vi "control daq.vi"(0 "Camera Device  IN":T1, 1 "Image Device IN":cluster{"Image":T5, "errorImage":errorcluster}, 2 "DAQ Device IN":T3={"DAQ Fs (S/s)"=10000.0, "task"="", "error"={"status"=FALSE, "code"=0, "source"=""}, "Min Value"=-10.0, "Max Value"=10.0}, 3 "Time Control Parameters":cluster{"# samples":u32, "tiempos (ms)":dbl}, 4 "Parametros Maximos":T6, 5 "detla Parametros":T6, 6 "Camara ON?":bool, 7 "Control Parameters":T4={"N Init Avg"=6, "N Avg Best"=3, "% Best to test"=0.95, "% Best to beat"=1.0}, 8 "Control?":bool=TRUE, 9 "Reset Control":bool, 10 "Ajuste?":bool=TRUE, 11 "Calibracion DAQ":T2) -> (14 "Camera Device OUT":T1, 15 "Image Device OUT":cluster{"Image":T5, "errorImage":errorcluster}, 16 "DAQ Device OUT":T3={"DAQ Fs (S/s)"=0.0, "task"="", "error"={"status"=FALSE, "code"=0, "source"=""}, "Min Value"=-10.0, "Max Value"=10.0}, 17 "Contraste":dbl, 18 "Waveform":waveform(dbl), 19 "Señal de Control":dbl[](array[numeric]))   [LabVIEW 2010]
uses:
  <vilib>/vision/Image Controls.llb/IMAQ Image.ctl
  <vilib>/measure/NI_MABase.lvlib
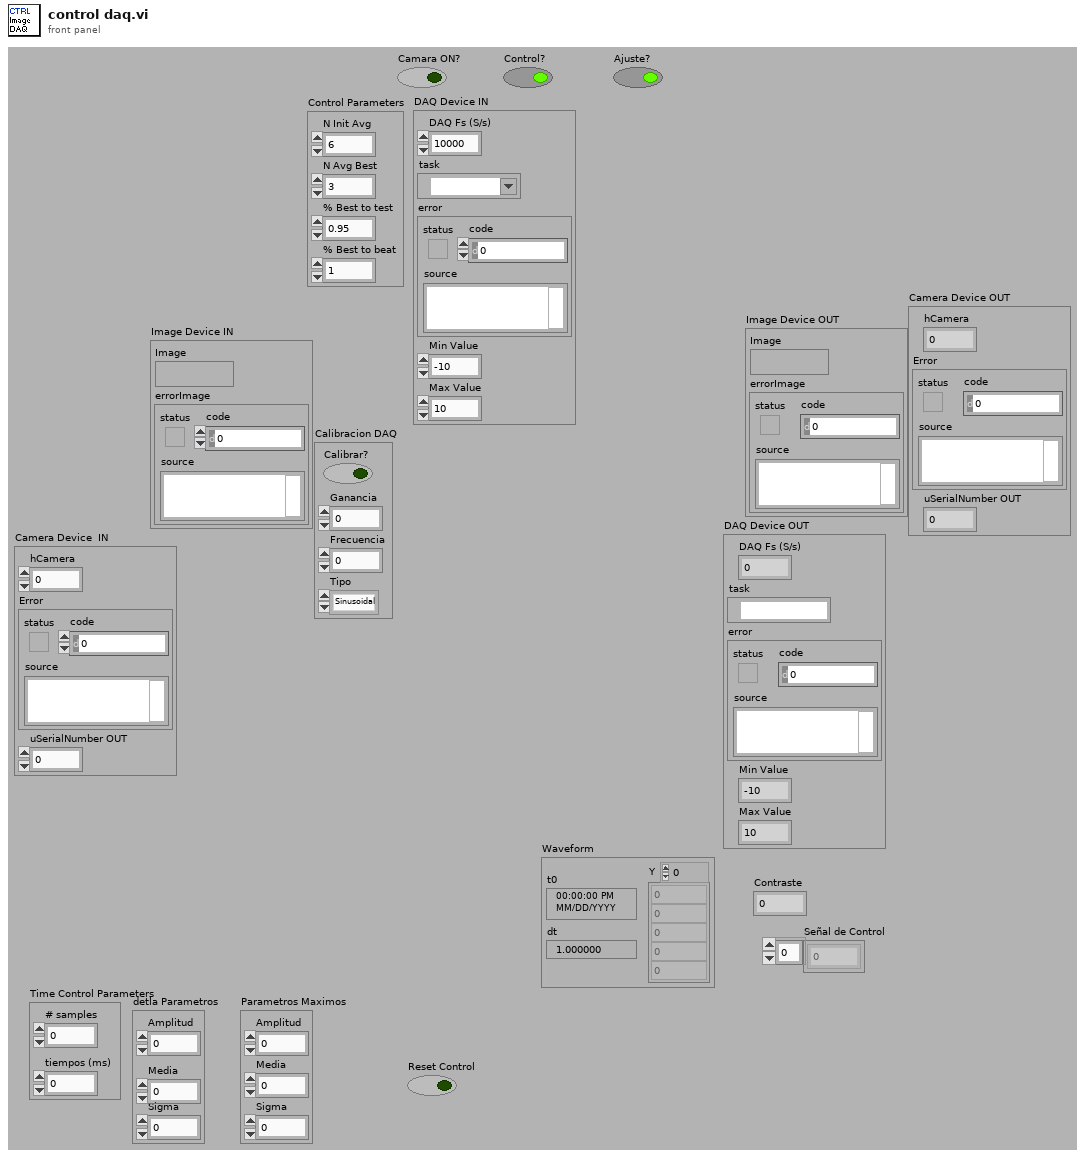
[diagram p1: front panel]
types:
  T1 = cluster{"hCamera":u32, "Error":errorcluster, "uSerialNumber OUT":u32}
  T2 = cluster{"Calibrar?":bool, "Ganancia":dbl, "Frecuencia":dbl, "Tipo":enum16{"Sinusoidal", "Triangular", "Cuadrada"}}
  T3 = cluster{"DAQ Fs (S/s)":dbl, "task":refnum<k21>, "error":errorcluster, "Min Value":dbl, "Max Value":dbl}
  T4 = cluster{"N Init Avg":u32, "N Avg Best":u32, "% Best to test":dbl, "% Best to beat":dbl}
  T5 = typedef "IMAQ Image.ctl" = refnum<image>
  T6 = cluster{"Amplitud":dbl, "Media":dbl, "Sigma":dbl}
  T7 = cluster{"DAQ Limits":cluster{"max":dbl, "min":dbl}, "Control Limits":cluster{"max":dbl, "min":dbl}}
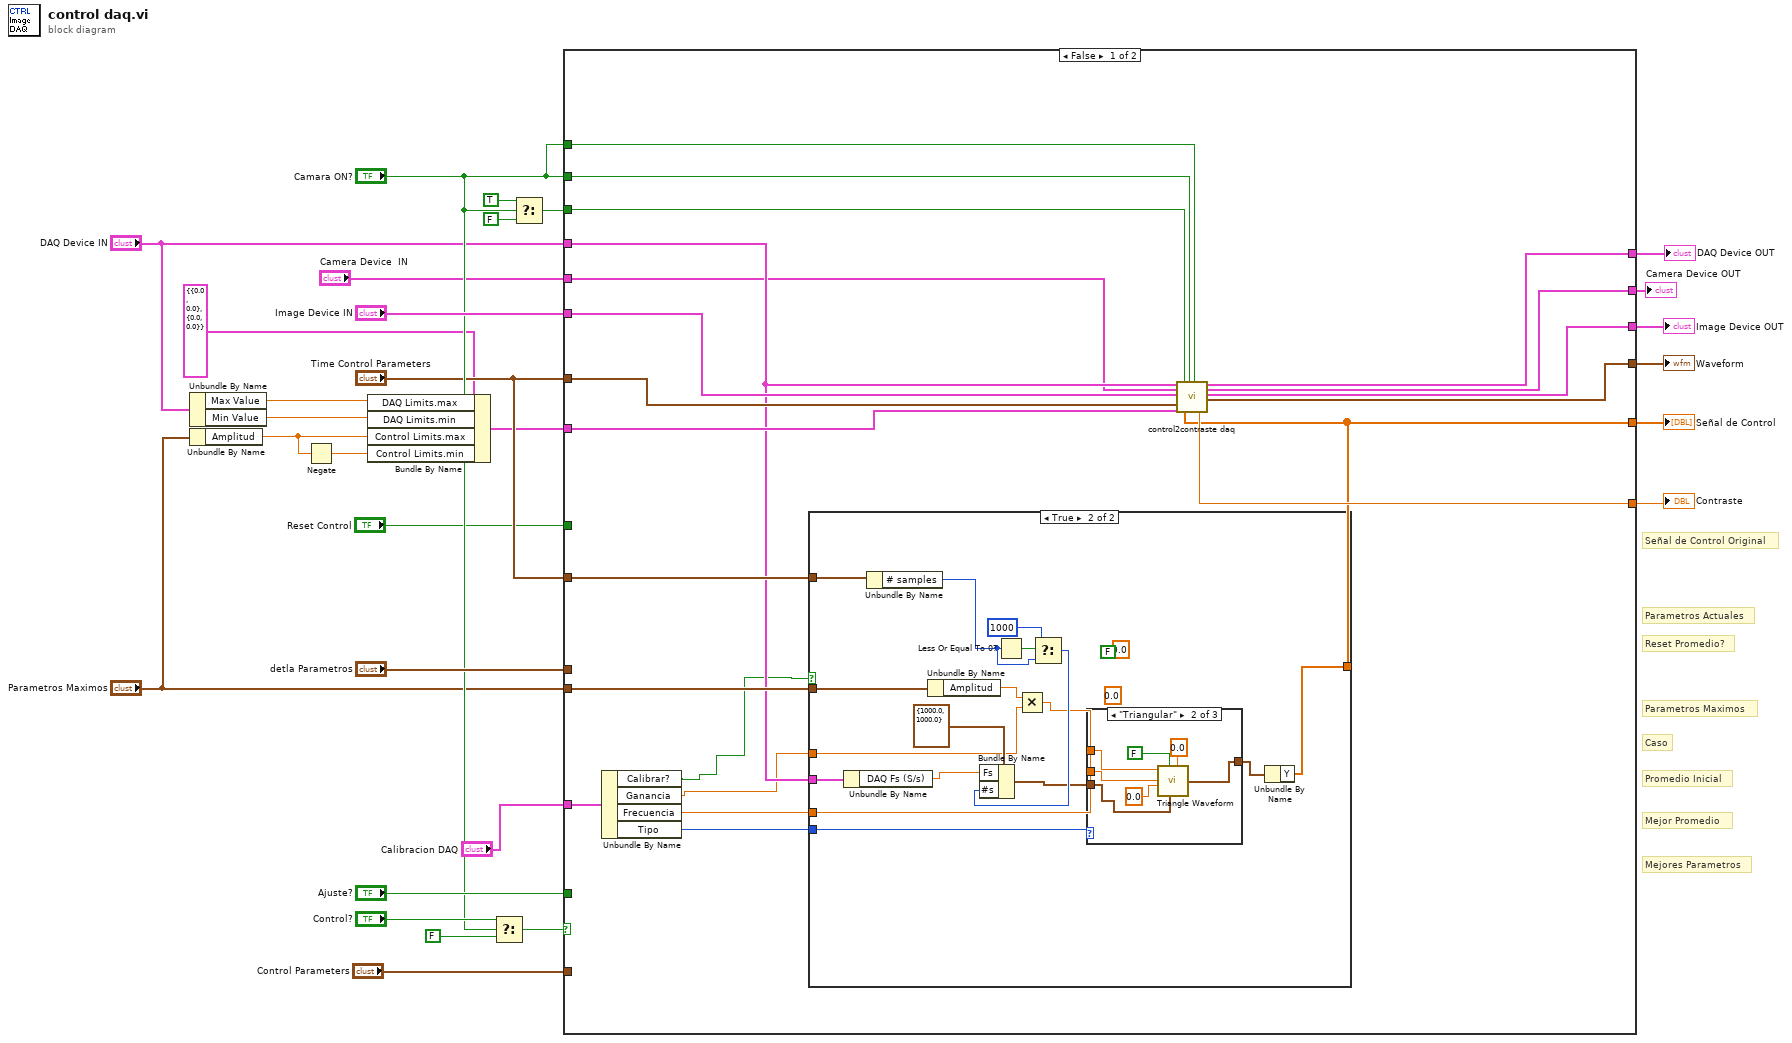
[diagram p0: block diagram]
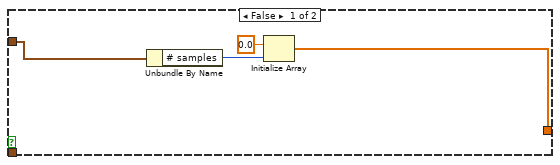
[diagram p2: hidden frame]
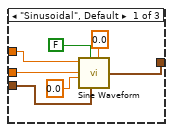
[diagram p3: hidden frame]
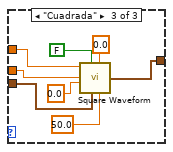
[diagram p4: hidden frame]
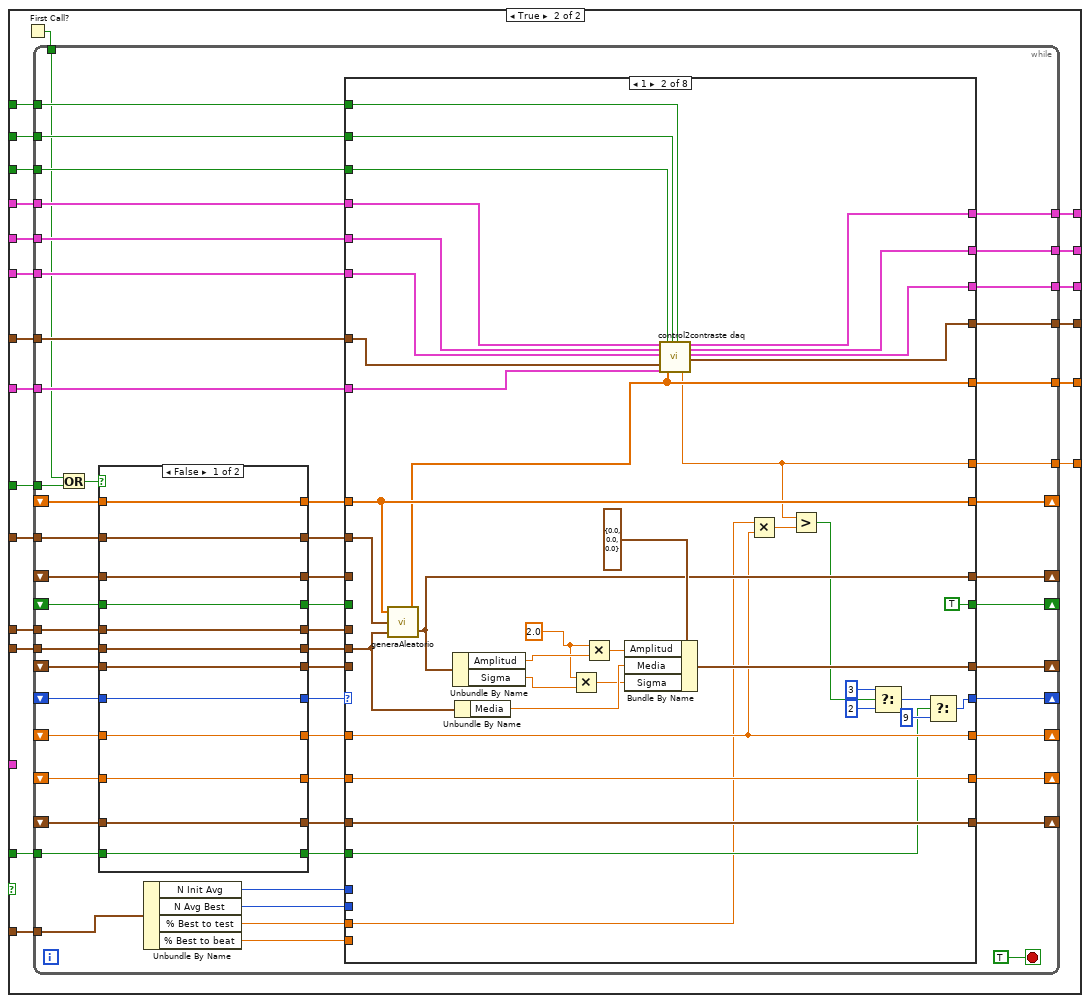
[diagram p5: hidden frame]
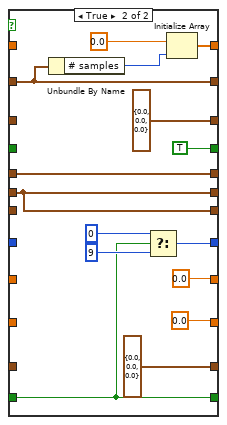
[diagram p6: hidden frame]
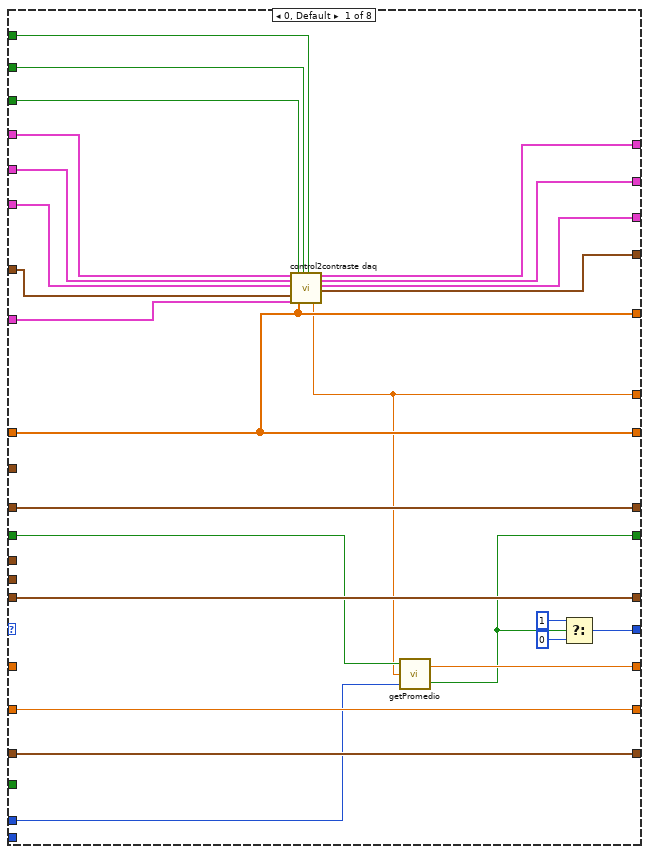
[diagram p7: hidden frame]
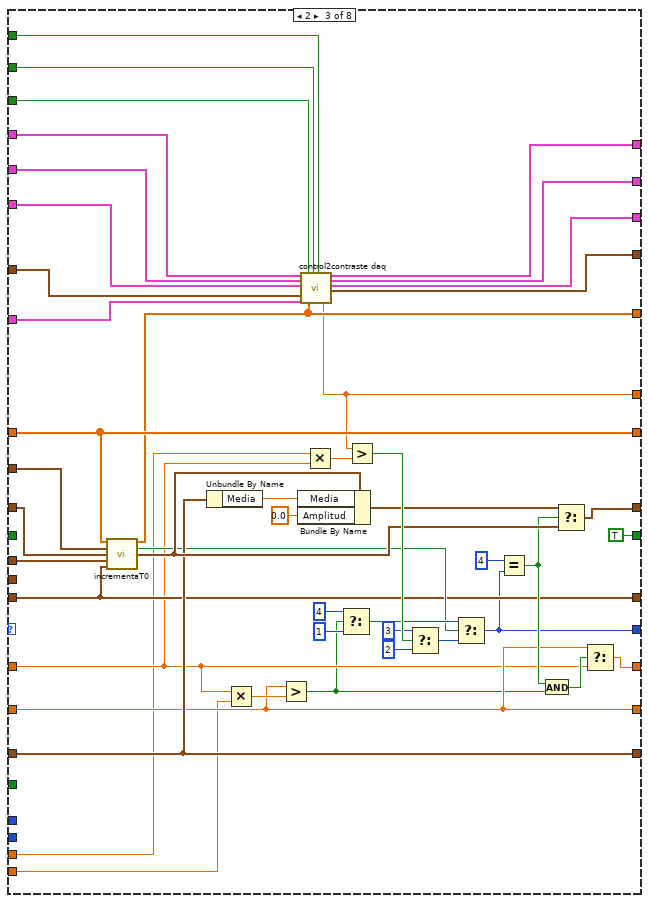
[diagram p8: hidden frame]
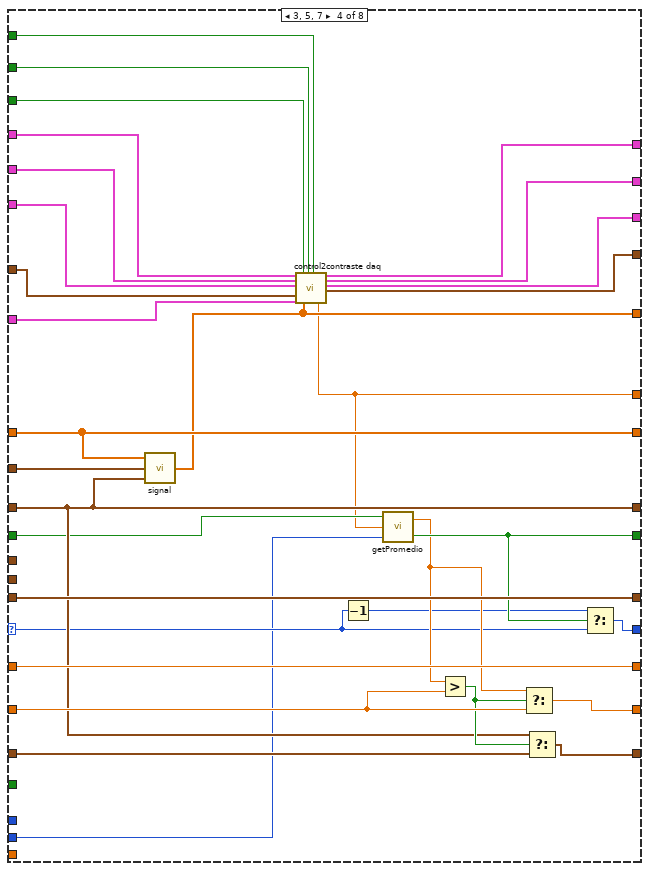
[diagram p9: hidden frame]
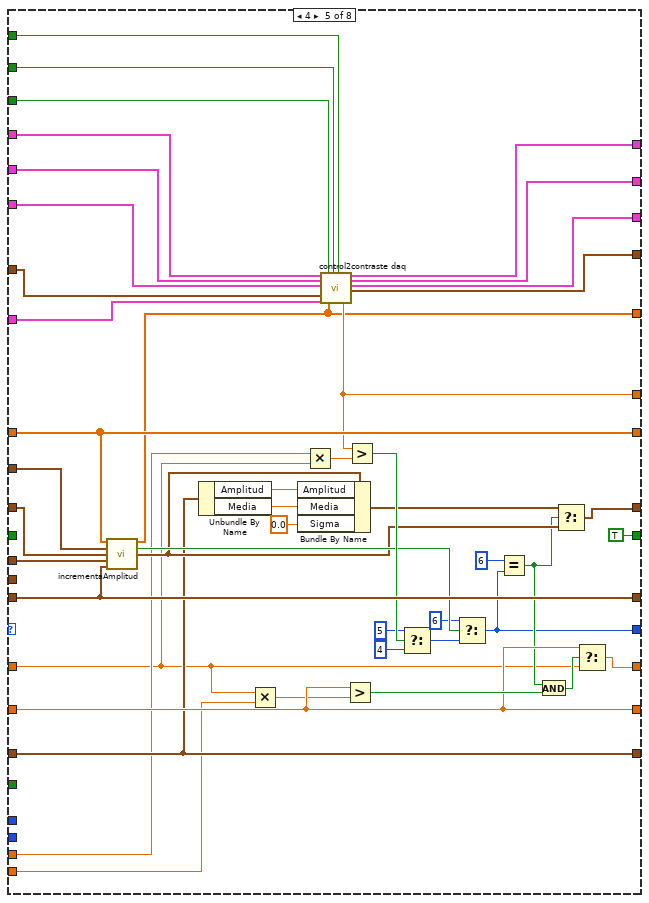
[diagram p10: hidden frame]
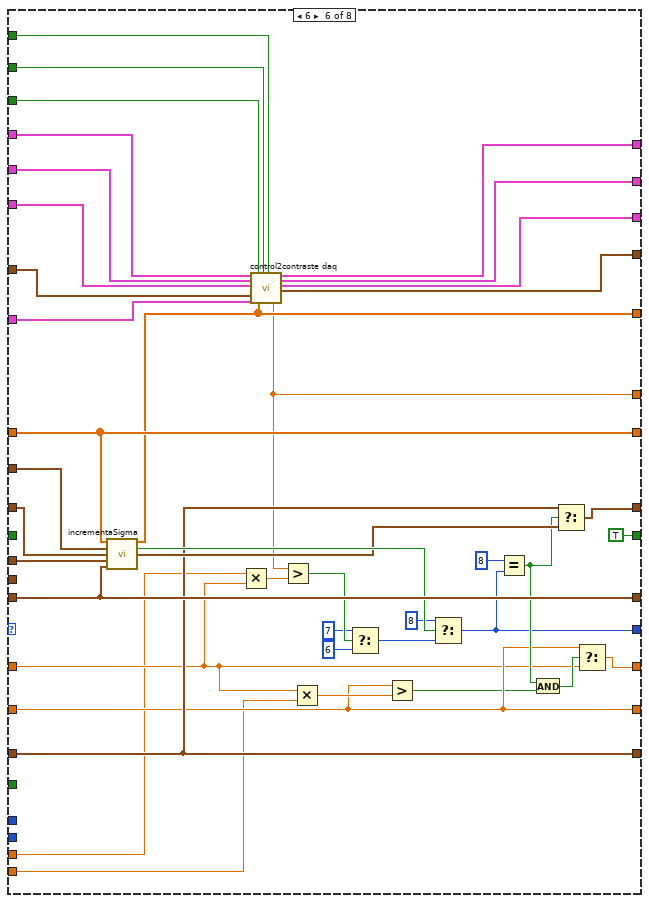
[diagram p11: hidden frame]
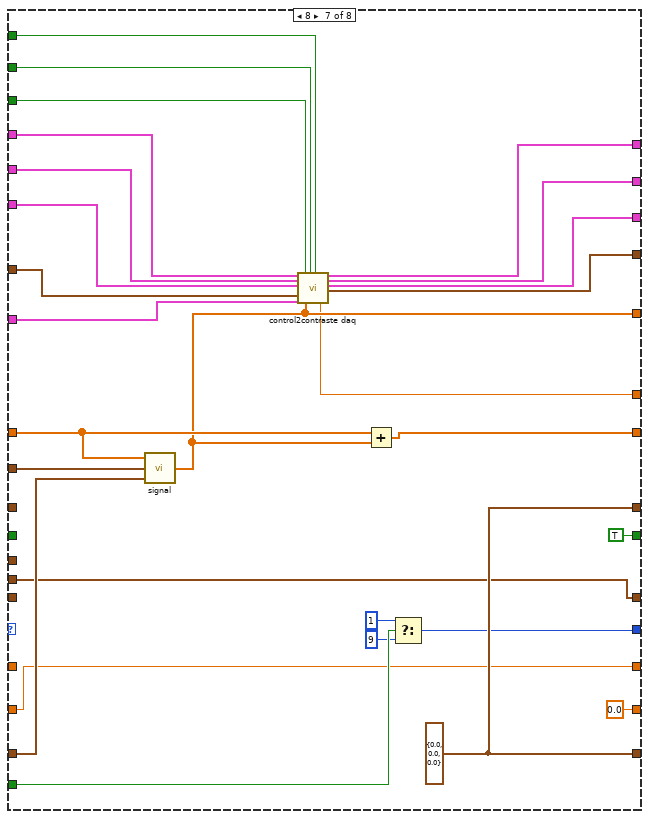
[diagram p12: hidden frame]
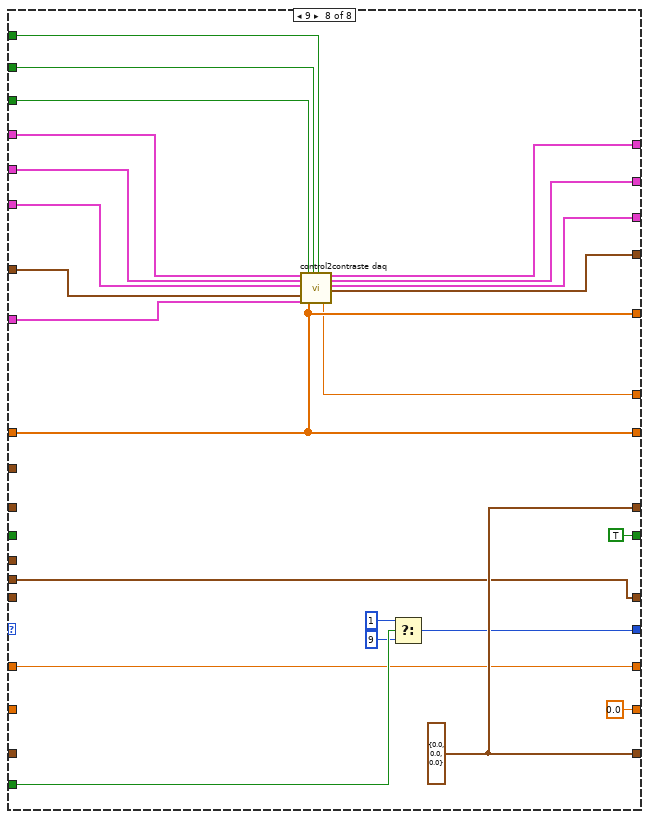
[diagram p13: hidden frame]
diagram:
  # "Reset Promedio?"
  # "Mejores Parametros"
  # "Mejor Promedio"
  # "Señal de Control Original"
  # "Parametros Actuales"
  # "Parametros Maximos"
  # "Caso"
  # "Promedio Inicial"
  n1 = Unbundle By Name("DAQ Device IN") -> ("Max Value"=w9:dbl, "Min Value"=w8:dbl)
  n2 = Unbundle By Name("Parametros Maximos") -> ("Amplitud"=w6:dbl)
  n3 = Negate(x=w6) -> (-x=w7:dbl)
  n4 = Bundle By Name(cluster=T7 {"DAQ Limits"={"max"=0.0, "min"=0.0}, "Control Limits"={"max"=0.0, "min"=0.0}} ("Limites"), "DAQ Limits.max"=w9, "DAQ Limits.min"=w8, "Control Limits.max"=w6, "Control Limits.min"=w7) -> (w10:T7)
  n5 = Select(t="Control?", s="Camara ON?", f=FALSE) -> (s? t:f=w19:bool)
  n6 = Select(t=TRUE, s="Camara ON?", f=FALSE) -> (s? t:f=w22:bool)
  n7 = case shown="False" w19 {
    tunnel: "Time Control Parameters" -> [w50 w114]
    tunnel: "detla Parametros" -> [_ w113]
    tunnel: "Parametros Maximos" -> [w38 w112]
    tunnel: "Ajuste?" -> [_ w110]
    tunnel: [w36 w109] -> w27
    tunnel: [w49 w108] -> w26
    tunnel: w10 -> [w48 w107]
    tunnel: "Time Control Parameters" -> [w47 w106]
    tunnel: "Image Device IN" -> [w46 w105]
    tunnel: "Camera Device  IN" -> [w30 w104]
    tunnel: "DAQ Device IN" -> [w37 w103]
    tunnel: w22 -> [w45 w102]
    tunnel: "Camara ON?" -> [w44 w101]
    tunnel: "Camara ON?" -> [w43 w100]
    tunnel: [w42 w99] -> w24
    tunnel: [w41 w98] -> w23
    tunnel: [w40 w97] -> w1
    tunnel: [w39 w96] -> w12
    tunnel: "Reset Control" -> [_ w95]
    tunnel: "Control Parameters" -> [_ w94]
    tunnel: "Calibracion DAQ" -> [w31 _]
    frame False {
      n8 = Unbundle By Name(w31) -> ("Calibrar?"=w35:bool, "Ganancia"=w34:dbl, "Frecuencia"=w33:dbl, "Tipo"=w32:enum16{"Sinusoidal", "Triangular", "Cuadrada"})
      n9 = case shown="True" w35 {
        tunnel: w50 -> [w52 w63]
        tunnel: w38 -> [_ w71]
        tunnel: w37 -> [_ w69]
        tunnel: [w51 w62] -> w36
        tunnel: w34 -> [_ w61]
        tunnel: w33 -> [_ w56]
        tunnel: w32 -> [_ w59]
        frame False {
          n10 = Unbundle By Name(w52) -> ("# samples"=w53:u32)
          n11 = Initialize Array(0.0 ("element"), w53) -> (w51:dbl[])
        }
        frame True {
          (unwired) FALSE ("reset signal")
          (unwired) 0.0 ("offset")
          (unwired) 0.0 ("phase")
          n12 = Unbundle By Name(w69) -> ("DAQ Fs (S/s)"=w68:dbl)
          n13 = Unbundle By Name(w63) -> ("# samples"=w64:u32)
          n14 = Unbundle By Name(w71) -> ("Amplitud"=w60:dbl)
          n15 = Less Or Equal To 0?(x=w64) -> (x <= 0?=w67:bool)
          n16 = Multiply(x=w60, y=w61) -> (x*y=w57:dbl)
          n17 = Select(t=u32 1000, s=w67, f=w64) -> (s? t:f=w65:u32)
          n18 = Bundle By Name(cluster=cluster{"Fs":dbl, "#s":dbl} {"Fs"=1000.0, "#s"=1000.0} ("sampling info"), "Fs"=w68, "#s"=w65) -> (w58:cluster{"Fs":dbl, "#s":dbl})
          n19 = case shown="\"Triangular\"" w59 {
            tunnel: w58 -> [w78 w80 w90]
            tunnel: w57 -> [w76 w81 w89]
            tunnel: w56 -> [w75 w82 w88]
            tunnel: [w72 w79 w87] -> w55
            frame "Sinusoidal", Default {
              n20 = call <vilib>:"Sine Waveform.vi"("offset"=0.0, "sampling info"=w78, "reset signal"=FALSE, "phase"=0.0, "amplitude"=w76, "frequency"=w75) -> ("signal out"=w72:waveform(dbl))  [unwired: 4 in, 1 out]
            }
            frame "Triangular" {
              n21 = call <vilib>:"Triangle Waveform.vi"("offset"=0.0, "sampling info"=w80, "reset signal"=FALSE, "phase"=0.0, "amplitude"=w81, "frequency"=w82) -> ("signal out"=w79:waveform(dbl))  [unwired: 4 in, 1 out]
            }
            frame "Cuadrada" {
              n22 = call <vilib>:"Square Waveform.vi"("duty cycle (%)"=50.0, "offset"=0.0, "sampling info"=w90, "reset signal"=FALSE, "phase"=0.0, "amplitude"=w89, "frequency"=w88) -> ("signal out"=w87:waveform(dbl))  [unwired: 3 in, 1 out]
            }
          }
          n23 = Unbundle By Name(w55) -> ("Y"=w62:dbl[])
        }
      }
      n24 = call "control2contraste daq.vi"("DAQ Device IN"=w37, "Camera Device  IN"=w30, "Image Device IN"=w46, "Time Control Parameters"=w47, "Limites"=w48, "DAQ?"=w45, "ControlSignal"=w36, "Streeam?"=w44, "Mostrar?"=w43) -> ("Contraste"=w49:dbl, "DAQ Device OUT"=w39:T3, "Camera Device OUT"=w40:T1, "Image Device OUT"=w41:cluster{"Image":T5, "errorImage":errorcluster}, "Waveform"=w42:waveform(dbl))  [unwired: 6 in]
    }
    frame True {
      n25 = First Call?() -> (First Call?: T/F=w111:bool)
      n26 = while {
        shift-right: [w166] -> _
        shift-left: _ -> [w153]
        tunnel: w114 -> [w145]
        shift-right: [w169] -> _
        shift-left: _ -> [w161]
        shift-right: [w168] -> _
        shift-left: _ -> [w155]
        shift-right: [w167] -> _
        shift-left: _ -> [w159]
        shift-right: [w165] -> _
        shift-left: _ -> [w151]
        tunnel: w113 -> [w142]
        shift-right: [w164] -> _
        shift-left: _ -> [w149]
        shift-right: [w163] -> _
        shift-left: _ -> [w147]
        shift-right: [w162] -> _
        shift-left: _ -> [w157]
        tunnel: w110 -> [w144]
        tunnel: w112 -> [w143]
        tunnel: w111 -> [w122]
        tunnel: [w137] -> w109
        tunnel: [w136] -> w108
        tunnel: w107 -> [w135]
        tunnel: w106 -> [w134]
        tunnel: w105 -> [w133]
        tunnel: w104 -> [w132]
        tunnel: w103 -> [w131]
        tunnel: w102 -> [w130]
        tunnel: w101 -> [w129]
        tunnel: w100 -> [w128]
        tunnel: [w127] -> w99
        tunnel: [w126] -> w98
        tunnel: [w125] -> w97
        tunnel: [w124] -> w96
        tunnel: w95 -> [w120]
        tunnel: w94 -> [w119]
        stop <- TRUE stop-if-true
        n27 = Or(x=w122, y=w120) -> (x .or. y?=w121:bool)
        n28 = case shown="False" w121 {
          tunnel: w161 -> [w181 _]
          tunnel: [w181 w196] -> w160
          tunnel: [w180 T6 {"Amplitud"=0.0, "Media"=0.0, "Sigma"=0.0} ("Parametros Iniciales")] -> w158
          tunnel: w159 -> [w180 _]
          tunnel: w157 -> [w179 _]
          tunnel: [w179 TRUE] -> w156
          tunnel: w155 -> [w178 _]
          tunnel: [w178 w185] -> w154
          tunnel: w153 -> [w177 _]
          tunnel: [w177 w186] -> w152
          tunnel: w151 -> [w176 _]
          tunnel: [w176 0.0 ("Contraste Promedio")] -> w150
          tunnel: w149 -> [w175 _]
          tunnel: [w175 0.0 ("Contraste Promedio")] -> w148
          tunnel: w147 -> [w174 _]
          tunnel: [w174 T6 {"Amplitud"=0.0, "Media"=0.0, "Sigma"=0.0} ("Parametros Maximos")] -> w146
          tunnel: w145 -> [w173 w182]
          tunnel: w143 -> [w171 w185]
          tunnel: w144 -> [w170 w183]
          tunnel: [w171 w185] -> w141
          tunnel: [w172 w184] -> w140
          tunnel: w142 -> [w172 w184]
          tunnel: [w170 w183] -> w139
          tunnel: [w173 w182] -> w138
          frame False {
          }
          frame True {
            n29 = Unbundle By Name(w182) -> ("# samples"=w194:u32)
            n30 = Select(t=u32 0, s=w183, f=u32 9) -> (s? t:f=w186:u32)
            n31 = Initialize Array(0.0 ("element"), w194) -> (w196:dbl[])
          }
        }
        n32 = Unbundle By Name(w119) -> ("N Init Avg"=w118:u32, "N Avg Best"=w117:u32, "% Best to test"=w116:dbl, "% Best to beat"=w115:dbl)
        n33 = case shown="1" w152 {
          selector: w152 -> [_ _ _ w322 _ _ _ _]
          tunnel: w160 -> [w211 w259 w303 w336 w379 w420 w442 w464]
          tunnel: w138 -> [_ w260 w306 w337 w382 w423 w450 _]
          tunnel: w154 -> [w214 _ w285 w328 w378 w419 _ _]
          tunnel: [w211 w259 w303 w336 w379 w420 w441 w464] -> w169
          tunnel: [w214 w258 w285 w328 w378 w419 w438 w466] -> w168
          tunnel: [w215 w256 w293 w327 w368 w411 w447 w472] -> w167
          tunnel: [w221 w223 w268 w335 w345 w389 w439 w467] -> w166
          tunnel: [w216 w246 w297 w334 w373 w415 w440 w465] -> w165
          tunnel: w150 -> [_ w246 w263 w334 w338 w385 _ w465]
          tunnel: [w210 w224 w283 w320 w359 w405 w436 w463] -> w136
          tunnel: [w211 w240 w284 w321 w358 w406 w437 w464] -> w137
          tunnel: w158 -> [w215 _ w305 w327 w381 w422 _ _]
          tunnel: w140 -> [_ _ w304 _ w380 w421 _ _]
          tunnel: [w217 w249 w265 w333 w371 w387 0.0 ("Contraste Promedio") 0.0 ("Contraste Promedio")] -> w164
          tunnel: [w218 w248 w290 w331 w365 w407 w447 w472] -> w163
          tunnel: w146 -> [w218 w248 w290 w329 w365 w407 w449 _]
          tunnel: w148 -> [w217 w249 w265 w332 w371 w387 w440 _]
          tunnel: w156 -> [w212 _ _ w326 _ _ _ _]
          tunnel: [w213 TRUE ("Llego a N?") TRUE ("Llego a N?") w325 TRUE ("Llego a N?") TRUE ("Llego a N?") TRUE ("Llego a N?") TRUE ("Llego a N?")] -> w162
          tunnel: w139 -> [_ w225 _ _ _ _ w445 w470]
          tunnel: w141 -> [_ w241 _ _ _ _ w438 w466]
          tunnel: w135 -> [w209 w239 w282 w319 w342 w404 w435 w462]
          tunnel: w134 -> [w208 w238 w281 w318 w343 w400 w434 w461]
          tunnel: w133 -> [w207 w237 w280 w317 w357 w399 w433 w460]
          tunnel: w132 -> [w206 w236 w279 w316 w356 w398 w432 w459]
          tunnel: w131 -> [w205 w228 w278 w315 w344 w397 w431 w458]
          tunnel: w130 -> [w204 w235 w277 w314 w355 w401 w430 w457]
          tunnel: w129 -> [w203 w234 w276 w313 w354 w402 w429 w456]
          tunnel: w128 -> [w202 w233 w275 w312 w353 w403 w428 w455]
          tunnel: [w201 w232 w274 w311 w352 w396 w427 w454] -> w127
          tunnel: [w200 w230 w273 w310 w351 w395 w426 w453] -> w126
          tunnel: [w199 w231 w272 w309 w350 w394 w425 w452] -> w125
          tunnel: [w198 w229 w271 w308 w349 w393 w424 w451] -> w124
          tunnel: w118 -> [w197 _ _ _ _ _ _ _]
          tunnel: w117 -> [_ _ _ w307 _ _ _ _]
          tunnel: w116 -> [_ w222 w261 _ w341 w384 _ _]
          tunnel: w115 -> [_ _ w264 _ w340 w386 _ _]
          frame 0, Default {
            n34 = call "control2contraste daq.vi"("DAQ Device IN"=w205, "Camera Device  IN"=w206, "Image Device IN"=w207, "Time Control Parameters"=w208, "Limites"=w209, "DAQ?"=w204, "ControlSignal"=w211, "Streeam?"=w203, "Mostrar?"=w202) -> ("Contraste"=w210:dbl, "DAQ Device OUT"=w198:T3, "Camera Device OUT"=w199:T1, "Image Device OUT"=w200:cluster{"Image":T5, "errorImage":errorcluster}, "Waveform"=w201:waveform(dbl))  [unwired: 6 in]
            n35 = call "getPromedio.vi"("N"=w197, "Contraste"=w210, "Reset"=w212) -> ("Llego a N?"=w213:bool, "Contraste Promedio"=w216:dbl)
            n36 = Select(t=u32 1, s=w213, f=u32 0) -> (s? t:f=w221:u32)
          }
          frame 1 {
            w251 = 2.0 ("x")
            n37 = call "generaAleatorio.vi"("Parametros Maximos"=w241, "Sound Parameters"=w260, "Señal de Control IN"=w259) -> ("Parametros Iniciales"=w256:T6, "Out"=w240:dbl[])
            n38 = Unbundle By Name(w256) -> ("Amplitud"=w255:dbl, "Sigma"=w252:dbl)
            n39 = Unbundle By Name(w241) -> ("Media"=w253:dbl)
            n40 = Multiply(x=w251, y=w252) -> (x*y=w250:dbl)
            n41 = Multiply(x=w251, y=w255) -> (x*y=w254:dbl)
            n42 = Bundle By Name(cluster=T6 {"Amplitud"=0.0, "Media"=0.0, "Sigma"=0.0} ("Parametros Iniciales"), "Amplitud"=w254, "Media"=w253, "Sigma"=w250) -> (w258:T6)
            n43 = call "control2contraste daq.vi"("DAQ Device IN"=w228, "Camera Device  IN"=w236, "Image Device IN"=w237, "Time Control Parameters"=w238, "Limites"=w239, "DAQ?"=w235, "ControlSignal"=w240, "Streeam?"=w234, "Mostrar?"=w233) -> ("Contraste"=w224:dbl, "DAQ Device OUT"=w229:T3, "Camera Device OUT"=w231:T1, "Image Device OUT"=w230:cluster{"Image":T5, "errorImage":errorcluster}, "Waveform"=w232:waveform(dbl))  [unwired: 6 in]
            n44 = Multiply(x=w222, y=w246) -> (x*y=w247:dbl)
            n45 = Greater?(x=w224, y=w247) -> (0:w245:bool)
            n46 = Select(t=u32 3, s=w245, f=u32 2) -> (s? t:f=w226:u32)
            n47 = Select(t=w226, s=w225, f=u32 9) -> (s? t:f=w223:u32)
          }
          frame 2 {
            n48 = call "incrementaT0.vi"("Señal de Control IN"=w303, "Sound Parameters"=w306, "Parametros Actuales IN"=w305, "detla Parametros"=w304, "Parametros Maximos"=w285) -> ("Out"=w284:dbl[], "Tope?"=w287:bool, "Parametros Actuales OUT"=w291:T6)  [unwired: 8 in]
            n49 = Unbundle By Name(w290) -> ("Media"=w289:dbl)
            n50 = Multiply(x=w263, y=w264) -> (x*y=w266:dbl)
            n51 = Greater?(x=w265, y=w266) -> (0:w262:bool)
            n52 = Bundle By Name(cluster=w291, "Media"=w289, "Amplitud"=0.0) -> (w292:T6)
            n53 = call "control2contraste daq.vi"("DAQ Device IN"=w278, "Camera Device  IN"=w279, "Image Device IN"=w280, "Time Control Parameters"=w281, "Limites"=w282, "DAQ?"=w277, "ControlSignal"=w284, "Streeam?"=w276, "Mostrar?"=w275) -> ("Contraste"=w283:dbl, "DAQ Device OUT"=w271:T3, "Camera Device OUT"=w272:T1, "Image Device OUT"=w273:cluster{"Image":T5, "errorImage":errorcluster}, "Waveform"=w274:waveform(dbl))  [unwired: 6 in]
            n54 = Multiply(x=w261, y=w263) -> (x*y=w302:dbl)
            n55 = Select(t=u32 4, s=w262, f=u32 1) -> (s? t:f=w298:u32)
            n56 = Greater?(x=w283, y=w302) -> (0:w301:bool)
            n57 = Select(t=u32 3, s=w301, f=u32 2) -> (s? t:f=w267:u32)
            n58 = Select(t=w298, s=w287, f=w267) -> (s? t:f=w268:u32)
            n59 = Equal?(x=u32 4, y=w268) -> (x = y?=w286:bool)
            n60 = And(x=w286, y=w262) -> (x .and. y?=w296:bool)
            n61 = Select(t=w292, s=w286, f=w291) -> (s? t:f=w293:T6)
            n62 = Select(t=w265, s=w296, f=w263) -> (s? t:f=w297:dbl)
          }
          frame 3, 5, 7 {
            n63 = call "signal.vi"("Parametros Actuales IN"=w327, "Sound Parameters"=w337, "Señal de Control IN"=w336) -> ("Out"=w321:dbl[])
            n64 = call "control2contraste daq.vi"("DAQ Device IN"=w315, "Camera Device  IN"=w316, "Image Device IN"=w317, "Time Control Parameters"=w318, "Limites"=w319, "DAQ?"=w314, "ControlSignal"=w321, "Streeam?"=w313, "Mostrar?"=w312) -> ("Contraste"=w320:dbl, "DAQ Device OUT"=w308:T3, "Camera Device OUT"=w309:T1, "Image Device OUT"=w310:cluster{"Image":T5, "errorImage":errorcluster}, "Waveform"=w311:waveform(dbl))  [unwired: 6 in]
            n65 = Decrement(x=w322) -> (x-1=w323:u32)
            n66 = call "getPromedio.vi"("N"=w307, "Contraste"=w320, "Reset"=w326) -> ("Llego a N?"=w325:bool, "Contraste Promedio"=w324:dbl)
            n67 = Greater?(x=w324, y=w332) -> (0:w330:bool)
            n68 = Select(t=w324, s=w330, f=w332) -> (s? t:f=w333:dbl)
            n69 = Select(t=w327, s=w330, f=w329) -> (s? t:f=w331:T6)
            n70 = Select(t=w323, s=w325, f=w322) -> (s? t:f=w335:u32)
          }
          frame 4 {
            n71 = call "incrementaAmplitud.vi"("Señal de Control IN"=w379, "Sound Parameters"=w382, "Parametros Actuales IN"=w381, "detla Parametros"=w380, "Parametros Maximos"=w378) -> ("Out"=w358:dbl[], "Tope?"=w375:bool, "Parametros Actuales OUT"=w366:T6)  [unwired: 8 in]
            n72 = Unbundle By Name(w365) -> ("Amplitud"=w364:dbl, "Media"=w362:dbl)
            n73 = Multiply(x=w338, y=w340) -> (x*y=w339:dbl)
            n74 = Bundle By Name(cluster=w366, "Amplitud"=w364, "Media"=w362, "Sigma"=0.0 ("Amplitud")) -> (w367:T6)
            n75 = Multiply(x=w341, y=w338) -> (x*y=w377:dbl)
            n76 = call "control2contraste daq.vi"("DAQ Device IN"=w344, "Camera Device  IN"=w356, "Image Device IN"=w357, "Time Control Parameters"=w343, "Limites"=w342, "DAQ?"=w355, "ControlSignal"=w358, "Streeam?"=w354, "Mostrar?"=w353) -> ("Contraste"=w359:dbl, "DAQ Device OUT"=w349:T3, "Camera Device OUT"=w350:T1, "Image Device OUT"=w351:cluster{"Image":T5, "errorImage":errorcluster}, "Waveform"=w352:waveform(dbl))  [unwired: 6 in]
            n77 = Greater?(x=w371, y=w339) -> (0:w374:bool)
            n78 = Greater?(x=w359, y=w377) -> (0:w376:bool)
            n79 = Select(t=u32 5, s=w376, f=u32 4) -> (s? t:f=w346:u32)
            n80 = Select(t=u32 6, s=w375, f=w346) -> (s? t:f=w345:u32)
            n81 = Equal?(x=u32 6, y=w345) -> (x = y?=w360:bool)
            n82 = And(x=w360, y=w374) -> (x .and. y?=w372:bool)
            n83 = Select(t=w367, s=w360, f=w366) -> (s? t:f=w368:T6)
            n84 = Select(t=w371, s=w372, f=w338) -> (s? t:f=w373:dbl)
          }
          frame 6 {
            n85 = call "incrementaSigma.vi"("Señal de Control IN"=w420, "Sound Parameters"=w423, "Parametros Actuales IN"=w422, "detla Parametros"=w421, "Parametros Maximos"=w419) -> ("Out"=w406:dbl[], "Tope?"=w416:bool, "Parametros Actuales OUT"=w410:T6)  [unwired: 8 in]
            n86 = Multiply(x=w384, y=w385) -> (x*y=w418:dbl)
            n87 = call "control2contraste daq.vi"("DAQ Device IN"=w397, "Camera Device  IN"=w398, "Image Device IN"=w399, "Time Control Parameters"=w400, "Limites"=w404, "DAQ?"=w401, "ControlSignal"=w406, "Streeam?"=w402, "Mostrar?"=w403) -> ("Contraste"=w405:dbl, "DAQ Device OUT"=w393:T3, "Camera Device OUT"=w394:T1, "Image Device OUT"=w395:cluster{"Image":T5, "errorImage":errorcluster}, "Waveform"=w396:waveform(dbl))  [unwired: 6 in]
            n88 = Greater?(x=w405, y=w418) -> (0:w417:bool)
            n89 = Multiply(x=w385, y=w386) -> (x*y=w388:dbl)
            n90 = Select(t=u32 7, s=w417, f=u32 6) -> (s? t:f=w390:u32)
            n91 = Greater?(x=w387, y=w388) -> (0:w383:bool)
            n92 = Select(t=u32 8, s=w416, f=w390) -> (s? t:f=w389:u32)
            n93 = Equal?(x=u32 8, y=w389) -> (x = y?=w408:bool)
            n94 = And(x=w408, y=w383) -> (x .and. y?=w414:bool)
            n95 = Select(t=w407, s=w408, f=w410) -> (s? t:f=w411:T6)
            n96 = Select(t=w387, s=w414, f=w385) -> (s? t:f=w415:dbl)
          }
          frame 8 {
            w447 = T6 {"Amplitud"=0.0, "Media"=0.0, "Sigma"=0.0} ("Parametros Maximos")
            n97 = call "signal.vi"("Parametros Actuales IN"=w449, "Sound Parameters"=w450, "Señal de Control IN"=w442) -> ("Out"=w437:dbl[])
            n98 = call "control2contraste daq.vi"("DAQ Device IN"=w431, "Camera Device  IN"=w432, "Image Device IN"=w433, "Time Control Parameters"=w434, "Limites"=w435, "DAQ?"=w430, "ControlSignal"=w437, "Streeam?"=w429, "Mostrar?"=w428) -> ("Contraste"=w436:dbl, "DAQ Device OUT"=w424:T3, "Camera Device OUT"=w425:T1, "Image Device OUT"=w426:cluster{"Image":T5, "errorImage":errorcluster}, "Waveform"=w427:waveform(dbl))  [unwired: 6 in]
            n99 = Add(x=w442, y=w437) -> (x+y=w441:dbl[])
            n100 = Select(t=u32 1, s=w445, f=u32 9) -> (s? t:f=w439:u32)
          }
          frame 9 {
            w472 = T6 {"Amplitud"=0.0, "Media"=0.0, "Sigma"=0.0} ("Parametros Maximos")
            n101 = call "control2contraste daq.vi"("DAQ Device IN"=w458, "Camera Device  IN"=w459, "Image Device IN"=w460, "Time Control Parameters"=w461, "Limites"=w462, "DAQ?"=w457, "ControlSignal"=w464, "Streeam?"=w456, "Mostrar?"=w455) -> ("Contraste"=w463:dbl, "DAQ Device OUT"=w451:T3, "Camera Device OUT"=w452:T1, "Image Device OUT"=w453:cluster{"Image":T5, "errorImage":errorcluster}, "Waveform"=w454:waveform(dbl))  [unwired: 6 in]
            n102 = Select(t=u32 1, s=w470, f=u32 9) -> (s? t:f=w467:u32)
          }
        }
      }
    }
  }
  "Señal de Control" <- w27
  "Contraste" <- w26
  "Image Device OUT" <- w23
  "Waveform" <- w24
  "DAQ Device OUT" <- w12
  "Camera Device OUT" <- w1
